vi "Read Visa com port.vi"(8 "error in (no error)":errorcluster, 11 "Serial device in":refnum<class "Serial device.lvclass">) -> (0 "error out":errorcluster, 2 "Visa com port":string, 3 "Serial device out":refnum<class "Serial device.lvclass">)   [LabVIEW 2020, in "Serial device.lvclass"]
doc: "Lee el puerto com con el que se trabaja"
uses:
  Serial device.lvclass
  Serial device.lvclass/Serial device.ctl
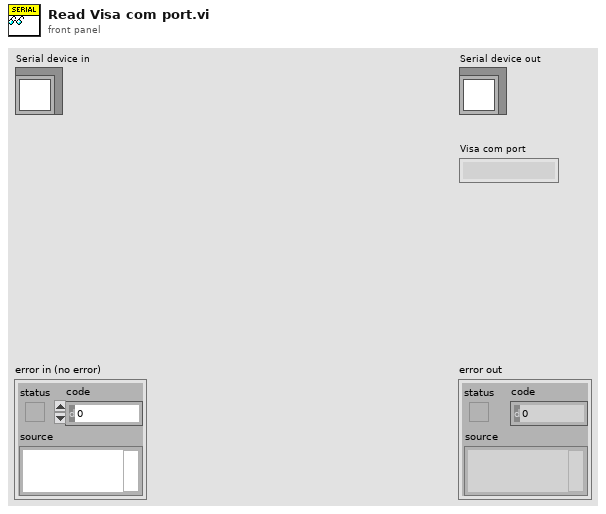
[diagram p1: front panel]
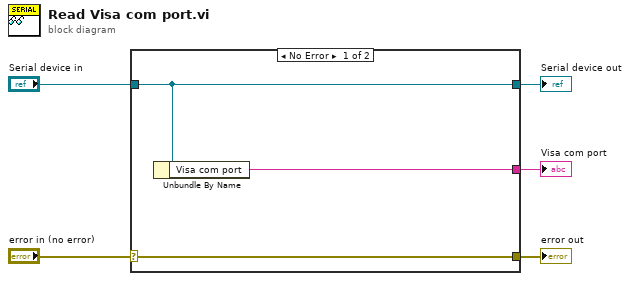
[diagram p0: block diagram]
diagram:
  n1 = case shown="No Error" "error in (no error)" {
    selector: "error in (no error)" -> [w8 w9]
    tunnel: [w8 w9] -> w4
    tunnel: [w7 w10] -> w2
    tunnel: "Serial device in" -> [w7 w10]
    tunnel: [w6 _] -> w1
    frame No Error {
      n2 = Unbundle By Name(w7) -> ("Visa com port"=w6:string)
    }
    frame Error {
    }
  }
  "error out" <- w4
  "Serial device out" <- w2
  "Visa com port" <- w1
